vi "Pv gen zen 42 test.vi"(0 "FluxStrIn":string, 1 "Numin":i32, 5 "errin":errorcluster, 6 "testlabel":string, 7 "Data limit":dbl[](array[numeric]), 8 "tab ref":string[][](array[string]), 10 "ligne à traiter":string[](array[string])) -> (14 "result string":string, 15 "Numout":i32, 19 "errout":errorcluster)   [LabVIEW 2017]
uses:
  <vilib>/regexp/Match Regular Expression.xnode
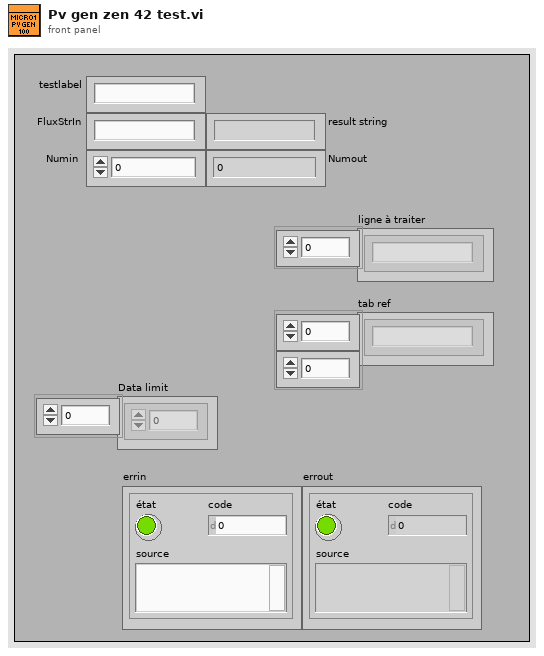
[diagram p1: front panel]
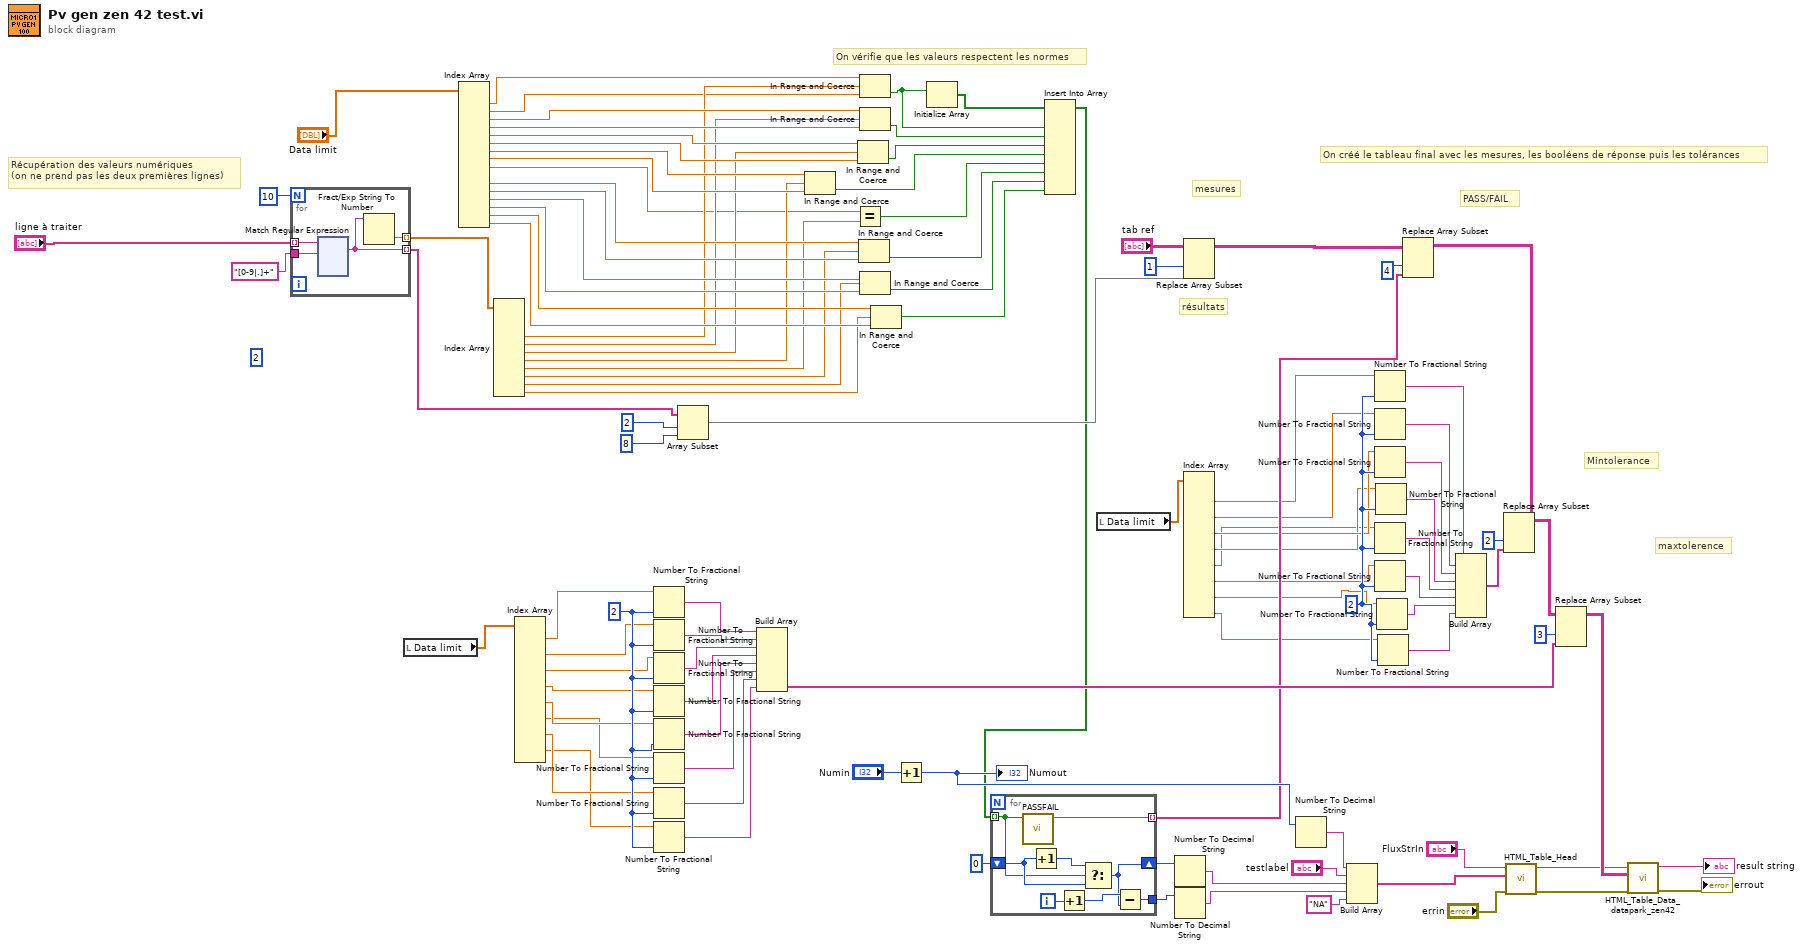
[diagram p0: block diagram]
diagram:
  (unwired) 2 ("indice")
  w40 = 2
  w50 = 2
  # "Récupération des valeurs numériques\n(on ne prend pas les deux premières lignes)"
  # "On créé le tableau final avec les mesures, les booléens de réponse puis les tolérances"
  # "On vérifie que les valeurs respectent les normes"
  # "maxtolerence"
  # "Mintolerance"
  # "mesures"
  # "PASS/FAIL"
  # "résultats"
  n1 = for {
    N: 10 -> [_]
    tunnel: "ligne à traiter" -> [w111] mode=indexing
    tunnel: "[0-9|.]+" ("expression régulière") -> [w110]
    tunnel: [w109] -> w5 mode=indexing
    tunnel: [w108] -> w4 mode=indexing
    n2 = xnode "Match Regular Expression"("input string"=w111, "regular expression"=w110) -> ("whole match"=w108:string)  [unwired: 4 in, 4 out]
    n3 = Fract/Exp String To Number(string=w108) -> (number=w109:dbl)  [unwired: 3 in, 1 out]
  }
  n4 = local read "Data limit"() -> (w31:dbl[])
  n5 = Index Array(array="Data limit") -> (element #1=w8:dbl, element #2=w7:dbl, element #3=w74:dbl, element #4=w73:dbl, element #5=w72:dbl, element #6=w71:dbl, element #7=w70:dbl, element #8=w69:dbl, element #9=w2:dbl, element #11=w68:dbl, element #12=w67:dbl, element #13=w66:dbl, element #14=w65:dbl, element #15=w64:dbl, element #16=w63:dbl)  [unwired: 16 in, 1 out]
  n6 = Index Array(array=w5) -> (element #3=w16:dbl, element #4=w17:dbl, element #5=w18:dbl, element #6=w19:dbl, element #7=w3:dbl, element #8=w20:dbl, element #9=w21:dbl, element #10=w22:dbl)  [unwired: 10 in, 2 out]
  n7 = Index Array(array=w31) -> (element #1=w30:dbl, element #3=w29:dbl, element #5=w28:dbl, element #7=w27:dbl, element #9=w26:dbl, element #11=w25:dbl, element #13=w24:dbl, element #15=w23:dbl)  [unwired: 16 in, 8 out]
  n8 = Number To Fractional String(number=w30, precision (6)=w40) -> (F-format string=w39:string)  [unwired: 2 in]
  n9 = Number To Fractional String(number=w29, precision (6)=w40) -> (F-format string=w38:string)  [unwired: 2 in]
  n10 = Number To Fractional String(number=w28, precision (6)=w40) -> (F-format string=w37:string)  [unwired: 2 in]
  n11 = Number To Fractional String(number=w27, precision (6)=w40) -> (F-format string=w36:string)  [unwired: 2 in]
  n12 = Number To Fractional String(number=w26, precision (6)=w40) -> (F-format string=w35:string)  [unwired: 2 in]
  n13 = Number To Fractional String(number=w25, precision (6)=w40) -> (F-format string=w34:string)  [unwired: 2 in]
  n14 = Number To Fractional String(number=w24, precision (6)=w40) -> (F-format string=w33:string)  [unwired: 2 in]
  n15 = Number To Fractional String(number=w23, precision (6)=w40) -> (F-format string=w32:string)  [unwired: 2 in]
  n16 = Array Subset(array=w4, index=2 ("indice"), length=8 ("longueur")) -> (w76:string[])
  n17 = Build Array(w39, w38, w37, w36, w35, w34, w33, w32) -> (w107:string[])
  n18 = In Range and Coerce(upper limit=w70, x=w19, lower limit=w69) -> (In Range?=w12:bool)  [unwired: 1 out]
  n19 = Equal?(x=w2, y=w3) -> (x = y?=w1:bool)
  n20 = In Range and Coerce(upper limit=w72, x=w18, lower limit=w71) -> (In Range?=w13:bool)  [unwired: 1 out]
  n21 = In Range and Coerce(upper limit=w68, x=w20, lower limit=w67) -> (In Range?=w11:bool)  [unwired: 1 out]
  n22 = In Range and Coerce(upper limit=w8, x=w16, lower limit=w7) -> (In Range?=w15:bool)  [unwired: 1 out]
  n23 = In Range and Coerce(upper limit=w74, x=w17, lower limit=w73) -> (In Range?=w14:bool)  [unwired: 1 out]
  n24 = In Range and Coerce(upper limit=w66, x=w21, lower limit=w65) -> (In Range?=w10:bool)  [unwired: 1 out]
  n25 = In Range and Coerce(upper limit=w64, x=w22, lower limit=w63) -> (In Range?=w9:bool)  [unwired: 1 out]
  n26 = Increment(x="Numin") -> (x+1=w93:i32)
  "Numout" <- w93
  n27 = Initialize Array(w15) -> (w62:bool[])  [unwired: 1 in]
  n28 = Insert Into Array(array=w62, new element #1=w15, new element #2=w14, new element #3=w13, new element #4=w12, new element #5=w1, new element #6=w11, new element #7=w10, new element #8=w9) -> (w59:bool[])  [unwired: 1 in]
  n29 = for {
    tunnel: w59 -> [w227] mode=indexing
    tunnel: [w226] -> w60 mode=indexing
    shift-right: [w229] -> w95
    shift-left: 0 -> [w232]
    tunnel: [w228] -> w96
    i -> [w231]
    n30 = call "PASSFAIL.vi"("E"=w227) -> ("S"=w226:string)  [unwired: 10 in]
    n31 = Increment(x=w232) -> (x+1=w233:i32)
    n32 = Increment(x=w231) -> (x+1=w230:i32)
    n33 = Select(t=w233, s=w227, f=w232) -> (s? t:f=w229:i32)
    n34 = Subtract(x=w230, y=w229) -> (x-y=w228:i32)
  }
  n35 = local read "Data limit"() -> (w49:dbl[])
  n36 = Number To Decimal String(number=w95) -> (decimal integer string=w97:string)  [unwired: 1 in]
  n37 = Number To Decimal String(number=w96) -> (decimal integer string=w98:string)  [unwired: 1 in]
  n38 = Replace Array Subset(array="tab ref", new element=w76, index (col)=1 ("indice désactivé (col)")) -> (w6:string[][])  [unwired: 1 in]
  n39 = Index Array(array=w49) -> (element #2=w48:dbl, element #4=w47:dbl, element #6=w46:dbl, element #8=w45:dbl, element #10=w44:dbl, element #12=w43:dbl, element #14=w42:dbl, element #16=w41:dbl)  [unwired: 16 in, 8 out]
  n40 = Number To Decimal String(number=w93) -> (decimal integer string=w81:string)  [unwired: 1 in]
  n41 = Build Array(w81, "testlabel", w97, w98, "NA" ("élément")) -> (w84:string[])
  n42 = Number To Fractional String(number=w48, precision (6)=w50) -> (F-format string=w51:string)  [unwired: 2 in]
  n43 = Number To Fractional String(number=w47, precision (6)=w50) -> (F-format string=w52:string)  [unwired: 2 in]
  n44 = Number To Fractional String(number=w46, precision (6)=w50) -> (F-format string=w53:string)  [unwired: 2 in]
  n45 = Number To Fractional String(number=w44, precision (6)=w50) -> (F-format string=w55:string)  [unwired: 2 in]
  n46 = Number To Fractional String(number=w43, precision (6)=w50) -> (F-format string=w56:string)  [unwired: 2 in]
  n47 = Number To Fractional String(number=w45, precision (6)=w50) -> (F-format string=w54:string)  [unwired: 2 in]
  n48 = Number To Fractional String(number=w42, precision (6)=w50) -> (F-format string=w57:string)  [unwired: 2 in]
  n49 = Number To Fractional String(number=w41, precision (6)=w50) -> (F-format string=w58:string)  [unwired: 2 in]
  n50 = Replace Array Subset(array=w6, new element=w60, index (col)=4 ("indice désactivé (col)")) -> (w101:string[][])  [unwired: 1 in]
  n51 = Build Array(w51, w52, w53, w54, w55, w56, w57, w58) -> (w106:string[])
  n52 = Replace Array Subset(array=w101, new element=w106, index (col)=2 ("indice désactivé (col)")) -> (w103:string[][])  [unwired: 1 in]
  n53 = call "HTML_Table_Head.vi"("entrée d'erreur (pas d'erreur)"="errin", "Tableau"=w84, "chaîne en entrée"="FluxStrIn") -> ("sortie d'erreur"=w83:errorcluster, "result string"=w82:string)  [unwired: 7 in]
  n54 = Replace Array Subset(array=w103, new element=w107, index (col)=3 ("indice désactivé (col)")) -> (w102:string[][])  [unwired: 1 in]
  n55 = call "HTML_Table_Data_datapark_zen42.vi"("entrée d'erreur (pas d'erreur)"=w83, "Tableau"=w102, "chaîne en entrée"=w82) -> ("sortie d'erreur"=→"errout":errorcluster, "result string"=→"result string":string)  [unwired: 7 in]
